vi "util.DO.FromString.vi"(9 "error in":errorcluster, 10 "initial string":string="1:3") -> (1 "error IO":errorcluster, 2 "output cluster":cluster{"state":bool, "timeoutSeconds":u16})   [LabVIEW 2024]
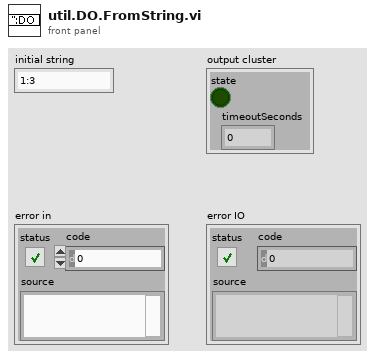
[diagram p1: front panel]
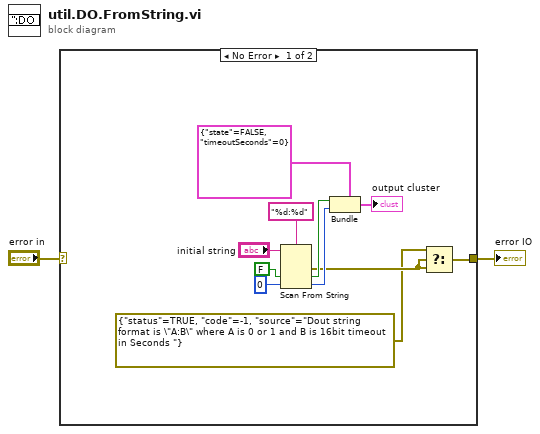
[diagram p0: block diagram]
diagram:
  n1 = case shown="No Error" "error in" {
    selector: "error in" -> [_ w14]
    tunnel: [w3 w14] -> w1
    frame No Error {
      n2 = Scan From String(format string="%d:%d", input string="initial string", default 1=FALSE ("state"), default 2=u16 0 ("timeoutSeconds")) -> (error out=w5:errorcluster, output 1=w10:bool, output 2=w9:u16)  [unwired: 2 in, 2 out]
      n3 = Bundle(cluster=cluster{"state":bool, "timeoutSeconds":u16} {"state"=FALSE, "timeoutSeconds"=0}, "state"=w10, "timeoutSeconds"=w9) -> (→"output cluster":cluster{"state":bool, "timeoutSeconds":u16})
      n4 = Select(t=errorcluster {"status"=TRUE, "code"=-1, "source"="Dout string format is \"A:B\" where A is 0 or 1 and B is 16bit timeout in Seconds "}, s=w5, f=w5) -> (s? t:f=w3:errorcluster)
    }
    frame Error {
    }
  }
  "error IO" <- w1
